vi "Password.vi"() -> ()   [LabVIEW 2015]
uses:
  Global/Globalclient.vi
panel:
  in  "quit":bool
  out "Message":string
  in  "OK":bool
  in  "Password":string="123456"
  in  "Username":string="admin"
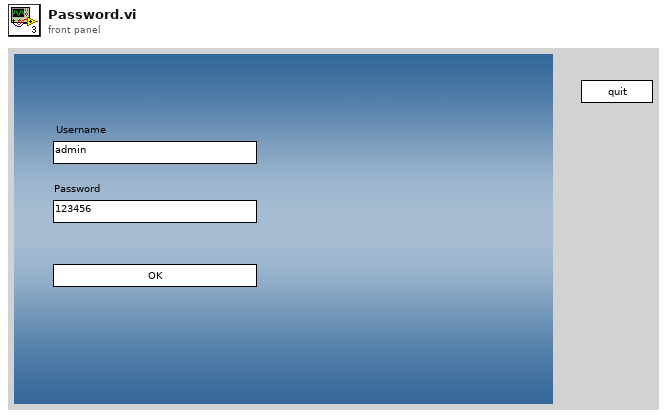
[diagram p1: front panel]
types:
  T1 = enum16{"Standard", "Buffered", "CRLF", "Immediate"}
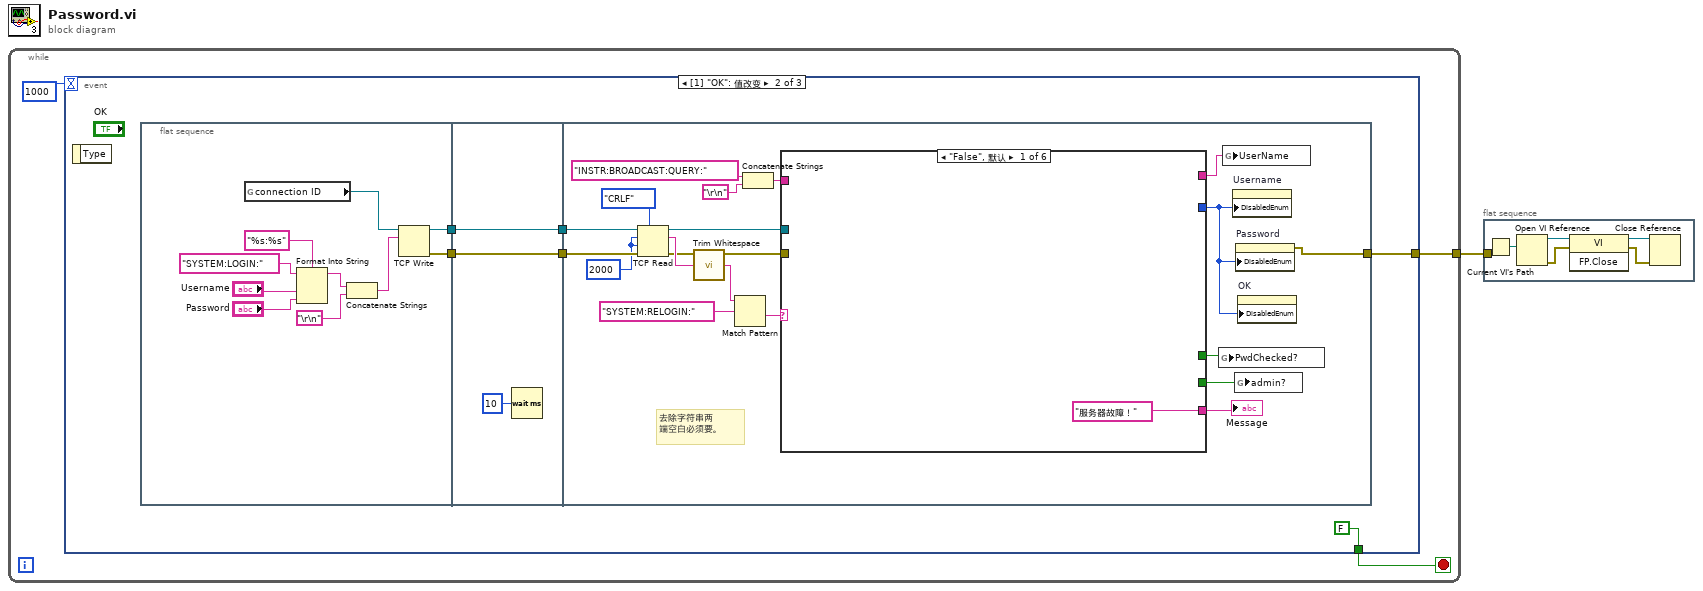
[diagram p0: block diagram]
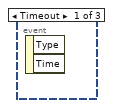
[diagram p2: hidden frame]
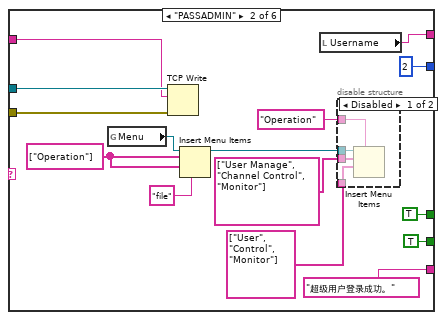
[diagram p3: hidden frame]
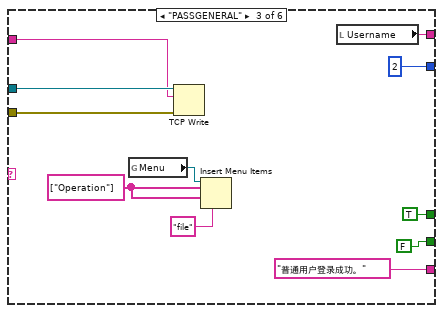
[diagram p5: hidden frame]
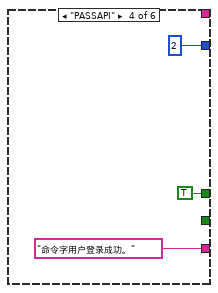
[diagram p6: hidden frame]
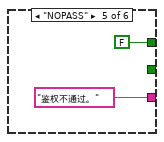
[diagram p7: hidden frame]
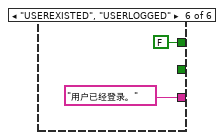
[diagram p8: hidden frame]
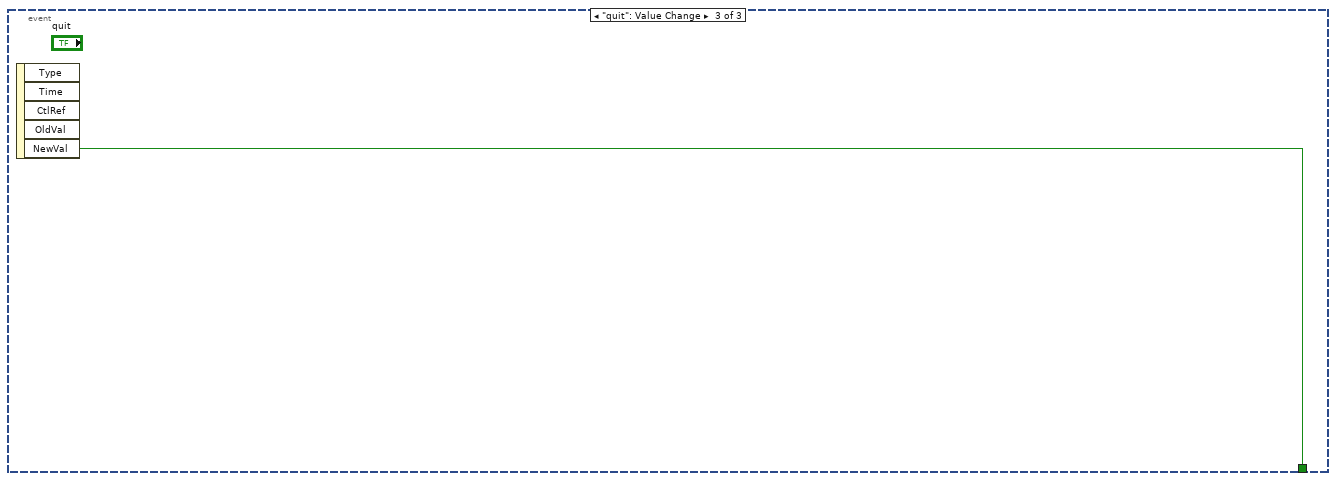
[diagram p9: hidden frame]
diagram:
  n1 = while {
    tunnel: [w2] -> w1
    stop <- w3 stop-if-true
    n2 = event shown="[1] \"OK\": 值改变" {
      selector: _ -> [_ _ _]
      dyn-events: _ -> [_ _ _]
      timeout: 1000 -> [_ _ _]
      tunnel: [_ FALSE w81] -> w3
      tunnel: [_ w6 _] -> w2
      event Timeout {
        n3 = event-data() -> ()  [unwired: 1 in, 2 out]
      }
      event "OK": Value Change {
        n4 = event-data() -> ()  [unwired: 1 in, 1 out]
        n5 = flat-sequence {
          tunnel: [w18] -> w10
          tunnel: [w17] -> w9
          tunnel: w10 -> [w22]
          tunnel: w9 -> [w21]
          tunnel: [w22] -> w8
          tunnel: [w21] -> w7
          tunnel: w8 -> [w42]
          tunnel: w7 -> [w41]
          tunnel: [w32] -> w6
          frame #0 {
            n6 = global read "Globalclient.vi" "connection ID"() -> (w16:refnum<k5>)
            n7 = Format Into String(format string="%s:%s", initial string="SYSTEM:LOGIN:", "Username", "Password") -> (resulting string=w11:string)  [unwired: 1 in, 1 out]
            n8 = Concatenate Strings(w11, "\r\n") -> (w19:string)
            n9 = TCP Write(connection ID=w16, data in=w19) -> (connection ID out=w18:refnum<k5>, error out=w17:errorcluster)  [unwired: 2 in, 1 out]
          }
          frame #1 {
            n10 = Wait (ms)(milliseconds to wait=u32 10 ("等待时间（毫秒）")) -> ()  [unwired: 1 out]
          }
          frame #2 {
            w39 = 2000 ("超时毫秒(25000)")
            # "去除字符串两\n端空白必须要。"
            n11 = TCP Read(connection ID=w42, bytes to read=w39, error in (no error)=w41, 7:T1."CRLF" ("mode (standard)"), 9:w39) -> (connection ID out=w31:refnum<k5>, data out=w35:string, error out=w30:errorcluster)
            n12 = call <vilib>:"Trim Whitespace.vi"("string"=w35) -> ("trimmed string"=w34:string)  [unwired: 1 in]
            n13 = Match Pattern(string=w34, regular expression="SYSTEM:RELOGIN:") -> (after substring=w37:string)  [unwired: 1 in, 3 out]
            n14 = Concatenate Strings("INSTR:BROADCAST:QUERY:", "\r\n") -> (w27:string)
            n15 = case shown="\"False\", 默认" w37 {
              tunnel: ["服务器故障！" "超级用户登录成功。" "普通用户登录成功。" "命令字用户登录成功。" "鉴权不通过。" "用户已经登录。"] -> w36
              tunnel: [_ 2 2 2 _ _] -> w33
              tunnel: [_ TRUE TRUE TRUE FALSE FALSE] -> w25
              tunnel: w31 -> [_ w48 w69 _ _ _]
              tunnel: w30 -> [_ w47 w68 _ _ _]
              tunnel: w27 -> [_ w46 w67 _ _ _]
              tunnel: [_ w45 w70 _ _ _] -> w26
              tunnel: [_ TRUE FALSE _ _ _] -> w24
              frame "False", Default {
              }
              frame "PASSADMIN" {
                w55 = string[] ["Operation"] ("项名称")
                n16 = global read "Globalclient.vi" "Menu"() -> (w57:refnum<k9>)
                n17 = TCP Write(connection ID=w48, data in=w46, error in (no error)=w47) -> ()  [unwired: 1 in, 3 out]
                n18 = Insert Menu Items(4:"file" ("项之后"), 7:w55, 8:w55, 9:w57) -> (3:w54:refnum<k9>)  [unwired: 2 in, 2 out]
                n19 = local read "Username"() -> (w45:string)
                n20 = disable-structure shown="Disabled" {
                  disable-tunnel: w54 -> [w62 _]
                  disable-tunnel: "Operation" -> [w61 _]
                  disable-tunnel: string[] ["User Manage", "Channel Control", "Monitor"] -> [w60 _]
                  disable-tunnel: string[] ["User", "Control", "Monitor"] -> [w59 _]
                  frame Disabled {
                    n21 = Insert Menu Items(5:w61, 7:w59, 8:w60, 9:w62) -> ()  [unwired: 2 in, 3 out]
                  }
                  frame Enabled {
                  }
                }
              }
              frame "PASSGENERAL" {
                w63 = string[] ["Operation"] ("项名称")
                n22 = global read "Globalclient.vi" "Menu"() -> (w65:refnum<k9>)
                n23 = TCP Write(connection ID=w69, data in=w67, error in (no error)=w68) -> ()  [unwired: 1 in, 3 out]
                n24 = Insert Menu Items(4:"file" ("项之后"), 7:w63, 8:w63, 9:w65) -> ()  [unwired: 2 in, 3 out]
                n25 = local read "Username"() -> (w70:string)
              }
              frame "PASSAPI" {
              }
              frame "NOPASS" {
              }
              frame "USEREXISTED", "USERLOGGED" {
              }
            }
            "Message" <- w36
            n26 = global write "Globalclient.vi" "PwdChecked?"(w25) -> ()
            n27 = global write "Globalclient.vi" "UserName"(w26) -> ()
            n28 = property on="Username" class="Str"("DisabledEnum"=w33) -> ()  [unwired: 2 in, 2 out]
            n29 = global write "Globalclient.vi" "admin?"(w24) -> ()
            n30 = property on="Password" class="Str"("DisabledEnum"=w33) -> (error out=w32:errorcluster)  [unwired: 2 in, 1 out]
            n31 = property on="OK" class="Bool"("DisabledEnum"=w33) -> ()  [unwired: 2 in, 2 out]
          }
        }
      }
      event "quit": Value Change {
        n32 = event-data() -> ("NewVal"=w81:bool)  [unwired: 1 in, 4 out]
      }
    }
  }
  n33 = flat-sequence {
    tunnel: w1 -> [_]
    frame #0 {
      n34 = Current VI's Path() -> (path=w86:path)
      n35 = Open VI Reference(vi path=w86) -> (vi reference=w83:refnum<vi>, error out=w82:errorcluster)  [unwired: 5 in]
      n36 = invoke class="VI" method="FP.Close"(reference=w83, error in=w82) -> (reference out=w85:refnum<vi>, error out=w84:errorcluster)  [unwired: 1 in, 1 out]
      n37 = Close Reference(reference=w85, error in (no error)=w84) -> ()  [unwired: 1 out]
    }
  }
